vi "_Generate DocMap.vi"(9 "Replace Ref(T)":bool=TRUE, 10 "Array 2":T2[](array[typedef]), 11 "Array":T1[](array[typedef])) -> (3 "Variant":variant)   [LabVIEW 2017, in "csmdoc.lvlib"]
uses:
  csmdoc.lvlib
  _Typedef/DocNote.ctl
  _Typedef/DocElement.ctl
  _Shared/CSM Shared.lvlib
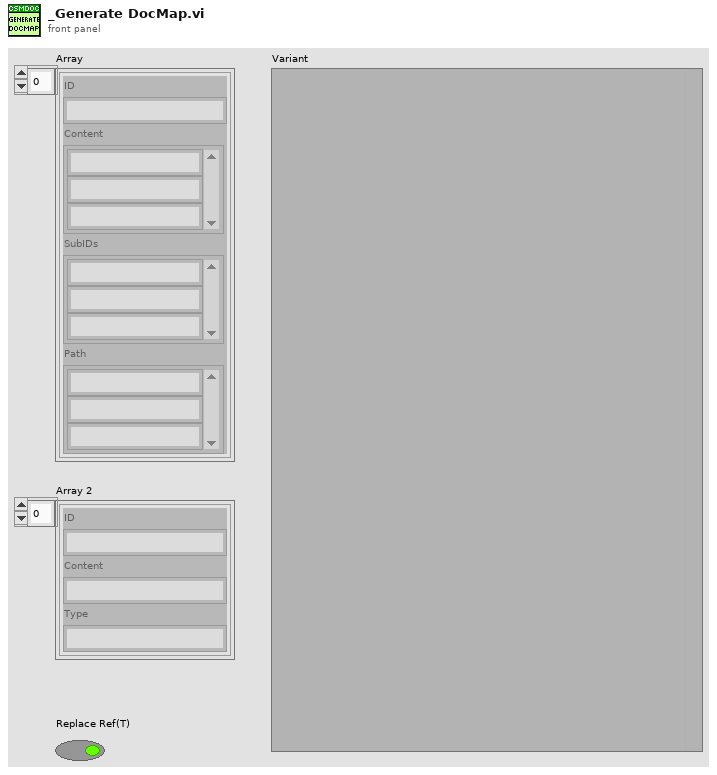
[diagram p1: front panel]
types:
  T1 = typedef "csmdoc.lvlib/DocElement.ctl" = cluster{"ID":string, "Content":string[], "SubIDs":string[], "Path":string[]}
  T2 = typedef "csmdoc.lvlib/DocNote.ctl" = cluster{"ID":string, "Content":string, "Type":string}
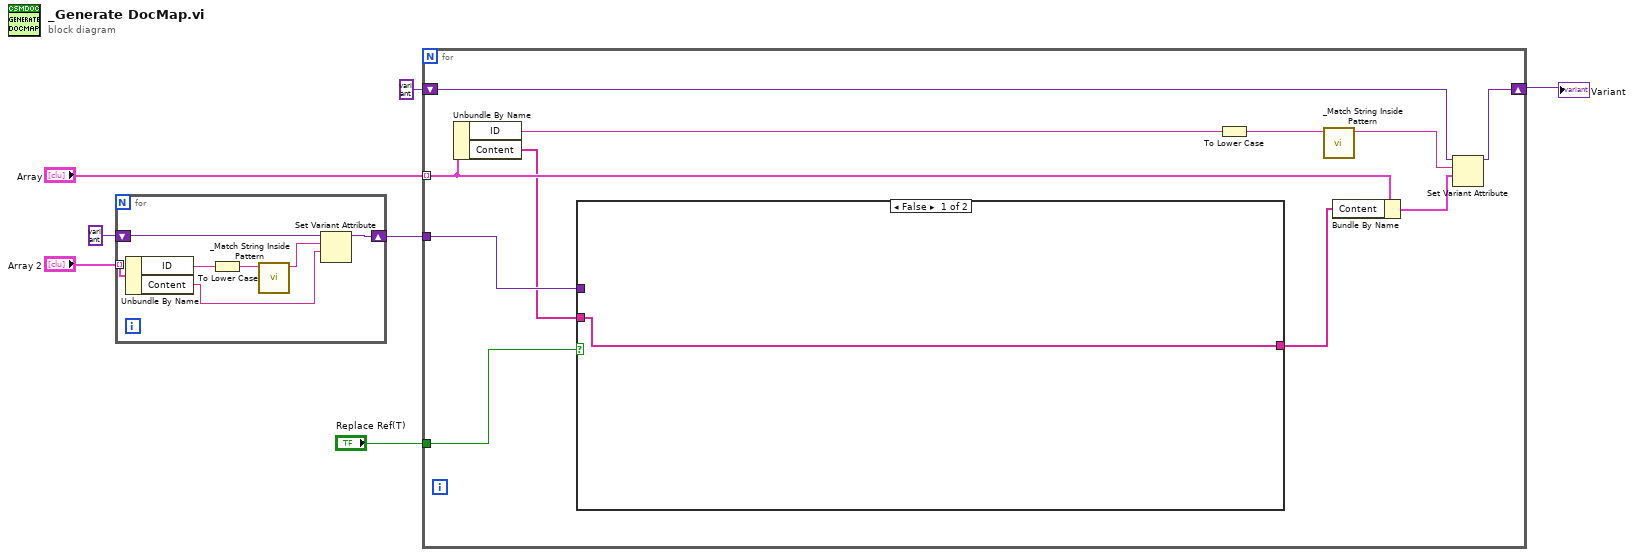
[diagram p0: block diagram]
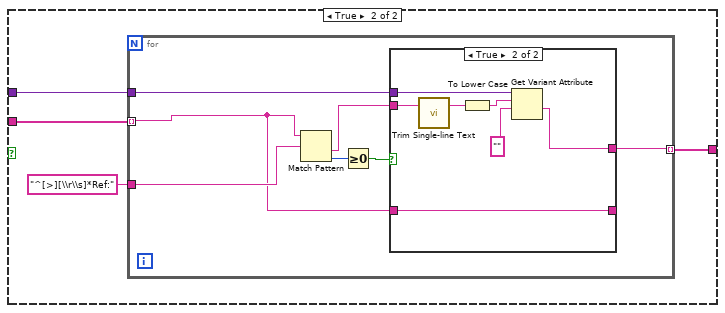
[diagram p2: hidden frame]
diagram:
  n1 = for {
    tunnel: "Array 2" -> [w12] mode=indexing
    shift-right: [w8] -> w2
    shift-left: variant -> [w14]
    n2 = Unbundle By Name(w12) -> ("ID"=w11:string, "Content"=w9:string)
    n3 = To Lower Case(string=w11) -> (all lower case string=w13:string)
    n4 = call "_Match String Inside Pattern.vi"("string"=w13) -> ("String inside"=w10:string)  [unwired: 10 in]
    n5 = Set Variant Attribute(Variant=w14, name=w10, value=w9) -> (Variant out=w8:variant)  [unwired: 1 in, 2 out]
  }
  n6 = for {
    tunnel: "Array" -> [w19] mode=indexing
    shift-right: [w24] -> w7
    shift-left: variant -> [w25]
    tunnel: w2 -> [w20]
    tunnel: "Replace Ref(T)" -> [w15]
    n7 = Unbundle By Name(w19) -> ("ID"=w23:string, "Content"=w16:string[])
    n8 = case shown="False" w15 {
      tunnel: w20 -> [_ w30]
      tunnel: [w26 w28] -> w18
      tunnel: w16 -> [w26 w27]
      frame False {
      }
      frame True {
        n9 = for {
          tunnel: w27 -> [w31] mode=indexing
          tunnel: w30 -> [w35]
          tunnel: "^[>][\\r\\s]*Ref:" ("delimited string") -> [w37]
          tunnel: [w32] -> w28 mode=indexing
          n10 = Match Pattern(string=w31, regular expression=w37) -> (after substring=w34:string, offset past match=w36:i32)  [unwired: 1 in, 2 out]
          n11 = Greater Or Equal To 0?(x=w36) -> (x >= 0?=w33:bool)
          n12 = case shown="True" w33 {
            tunnel: w35 -> [_ w45]
            tunnel: w34 -> [_ w43]
            tunnel: [w38 w40] -> w32
            tunnel: w31 -> [w38 w39]
            tunnel: [_ w39] -> _
            frame False {
            }
            frame True {
              n13 = call "Trim Single-line Text.vi"("single-line text"=w43) -> ("trimed text"=w42:string)  [unwired: 2 in]
              n14 = To Lower Case(string=w42) -> (all lower case string=w44:string)
              n15 = Get Variant Attribute(Variant=w45, name=w44, default value (empty Variant)="" ("delimited string")) -> (value=w40:string)  [unwired: 1 in, 3 out]
            }
          }
        }
      }
    }
    n16 = To Lower Case(string=w23) -> (all lower case string=w22:string)
    n17 = call "_Match String Inside Pattern.vi"("string"=w22) -> ("String inside"=w21:string)  [unwired: 10 in]
    n18 = Bundle By Name(cluster=w19, "Content"=w18) -> (w17:T1)
    n19 = Set Variant Attribute(Variant=w25, name=w21, value=w17) -> (Variant out=w24:variant)  [unwired: 1 in, 2 out]
  }
  "Variant" <- w7
